vi "Get environment variable.vi"(3 "Variable name":string) -> (1 "Value":string)   [LabVIEW 2015]
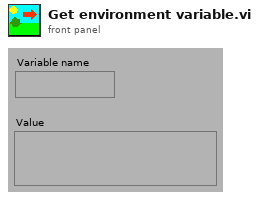
[diagram p1: front panel]
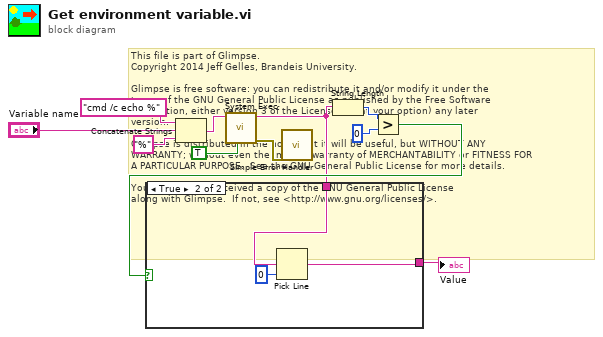
[diagram p0: block diagram]
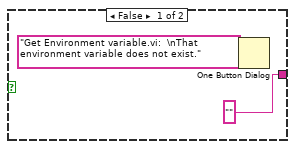
[diagram p2: hidden frame]
diagram:
  # "This file is part of Glimpse. \nCopyright 2014 Jeff Gelles, Brandeis University.    \n\nGlimpse is free software: you can redistribute it and/or modify it under the \nterms of the GNU General Public License as published by the Free Software \nFoundation, either version 3 of the License, or (at your option) any later \nversion.\n\nGlimpse is distributed in the hope that it will be useful, but WITHOUT ANY \nWARRANTY; without even the implied warranty of MERCHANTABILITY or FITNESS FOR \nA PARTICULAR PURPOSE.  See the GNU General Public License for more details.\n\nYou should have received a copy of the GNU General Public License\nalong with Glimpse.  If not, see <http://www.gnu.org/licenses/>."
  n1 = Concatenate Strings("cmd /c echo %", "Variable name", "%") -> (w2:string)
  n2 = call <vilib>:"System Exec.vi"("run minimized? (F)"=TRUE, "command line"=w2) -> ("error out"=w3:errorcluster, "standard output"=w4:string)  [unwired: 4 in, 4 out]
  n3 = call <vilib>:"Simple Error Handler.vi"("error in (no error)"=w3) -> ()  [unwired: 1 in, 8 out]
  n4 = String Length(string=w4) -> (length=w8:i32)
  n5 = Greater?(x=w8, y=0) -> (0:w5:bool)
  n6 = case shown="True" w5 {
    tunnel: ["" ("Command Output") w15] -> w6
    tunnel: w4 -> [_ w16]
    frame False {
      n7 = One Button Dialog(message="Get Environment variable.vi:  \nThat environment variable does not exist.") -> ()  [unwired: 2 out]
    }
    frame True {
      n8 = Pick Line(multi-line string=w16, line index=0) -> (output string=w15:string)  [unwired: 1 out]
    }
  }
  "Value" <- w6
